vi "lockin - Set REF f equal AO f.vi"(9 "REE = AO?":bool, 10 "Lockin":T1={"REF f (Hz)"=[13.0, 13.0, 13.0, 13.0, 13.0, 13.0, 13.0, 13.0], "REF phi (deg)"=[0.0, 0.0, 0.0, 0.0, 0.0, 0.0, 0.0, 0.0]} {"REF phi (deg)" format="%#_3g"}, 11 "AO":T2={"AO amp (V)"=[0.1, 0.09, 0.08, 0.07, 0.06, 0.05, 0.04, 0.03], "AO DC (V)"=[0.0, 0.0, 0.0, 0.0, 0.0, 0.0, 0.0, 0.0], "AO f (Hz)"=[13.0, 13.0, 13.0, 13.0, 13.0, 13.0, 13.0, 13.0], "AO phi (deg)"=[0.0, 0.0, 0.0, 0.0, 0.0, 0.0, 0.0, 0.0], "function"=[enum."Sine Wave", enum."Sine Wave", enum."Sine Wave", enum."Sine Wave", enum."Sine Wave", enum."Sine Wave", enum."Sine Wave", enum."Sine Wave"]} {"AO DC (V)" format="%#_6p"; "AO amp (V)" format="%#_6p"}) -> (2 "Lockin 2":T1={"REF f (Hz)"=[13.0, 13.0, 13.0, 13.0, 13.0, 13.0, 13.0, 13.0], "REF phi (deg)"=[0.0, 0.0, 0.0, 0.0, 0.0, 0.0, 0.0, 0.0]} {"REF phi (deg)" format="%#_3g"}, 3 "AO 2":T2={"AO amp (V)"=[0.1, 0.09, 0.08, 0.07, 0.06, 0.05, 0.04, 0.03], "AO DC (V)"=[0.0, 0.0, 0.0, 0.0, 0.0, 0.0, 0.0, 0.0], "AO f (Hz)"=[13.0, 13.0, 13.0, 13.0, 13.0, 13.0, 13.0, 13.0], "AO phi (deg)"=[0.0, 0.0, 0.0, 0.0, 0.0, 0.0, 0.0, 0.0], "function"=[enum."Sine Wave", enum."Sine Wave", enum."Sine Wave", enum."Sine Wave", enum."Sine Wave", enum."Sine Wave", enum."Sine Wave", enum."Sine Wave"]} {"AO DC (V)" format="%#_6p"; "AO amp (V)" format="%#_6p"})   [LabVIEW 2016, in "LockinDAQ.lvclass"]
uses:
  LockinDAQ.lvclass
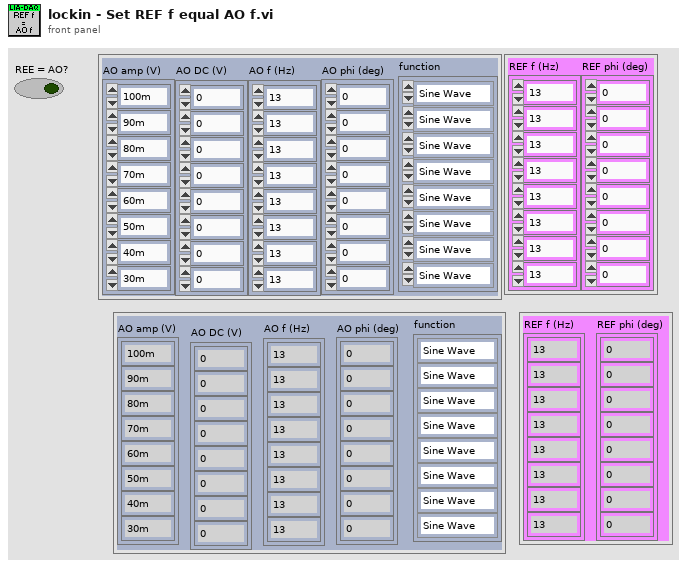
[diagram p1: front panel]
types:
  T1 = cluster{"REF f (Hz)":dbl[], "REF phi (deg)":dbl[]}
  T2 = cluster{"AO amp (V)":dbl[], "AO DC (V)":dbl[], "AO f (Hz)":dbl[], "AO phi (deg)":dbl[], "function":enum16{"Sine Wave", "Triangle Wave", "Square Wave", "Sawtooth Wave"}[]}
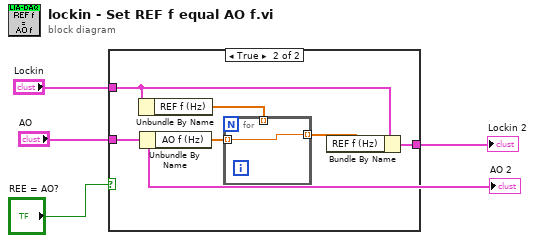
[diagram p0: block diagram]
diagram:
  n1 = case shown="True" "REE = AO?" {
    tunnel: "Lockin" -> [w5 w9]
    tunnel: "AO" -> [_ w11]
    tunnel: [w5 w10] -> w2
    frame False {
    }
    frame True {
      n2 = Unbundle By Name(w9) -> ("REF f (Hz)"=w8:dbl[])
      n3 = Unbundle By Name(w11) -> ("AO f (Hz)"=w6:dbl[])
      n4 = for {
        tunnel: w8 -> [_] mode=indexing
        tunnel: [w12] -> w7 mode=indexing
        tunnel: w6 -> [w12] mode=indexing
      }
      n5 = Bundle By Name(cluster=w9, "REF f (Hz)"=w7) -> (w10:T1)
    }
  }
  "Lockin 2" <- w2
  "AO 2" <- "AO"
